vi "test.Template.vi"(8 "error in":errorcluster, 10 "Data":variant, 11 "Command":string) -> (0 "error out":errorcluster, 3 "Return Data":variant)   [LabVIEW 2014]
uses:
  Private/Class/meth.Constructor.vi
  Private/Class/meth.Destructor.vi
  GLue.lvlib
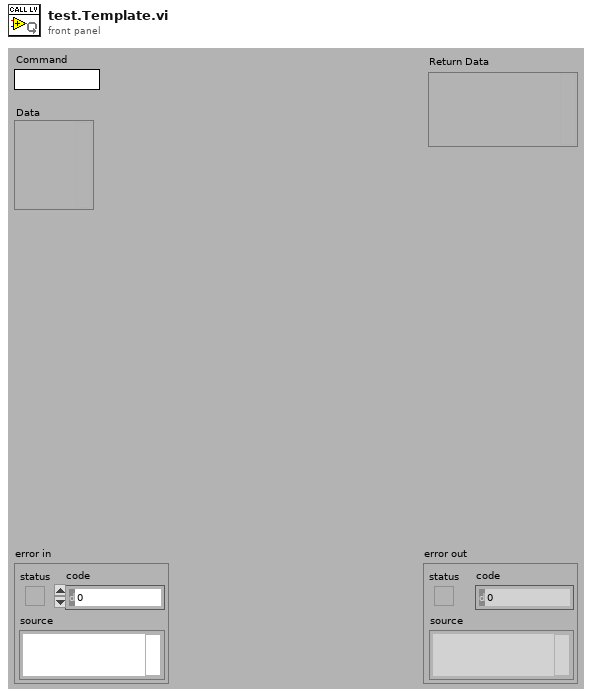
[diagram p1: front panel]
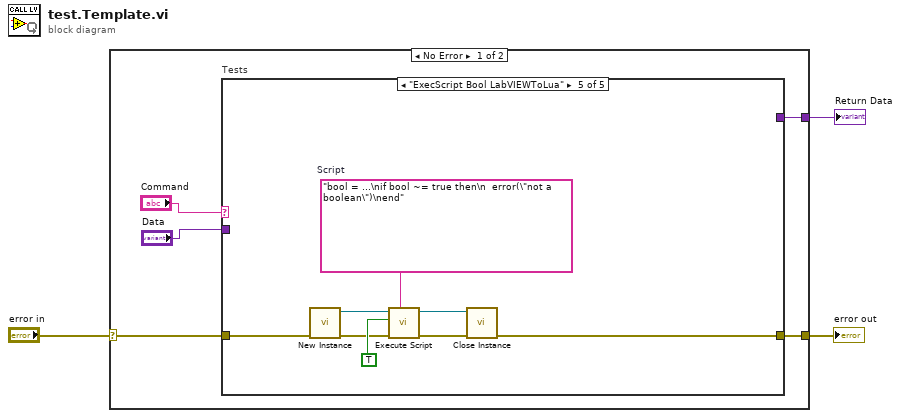
[diagram p0: block diagram]
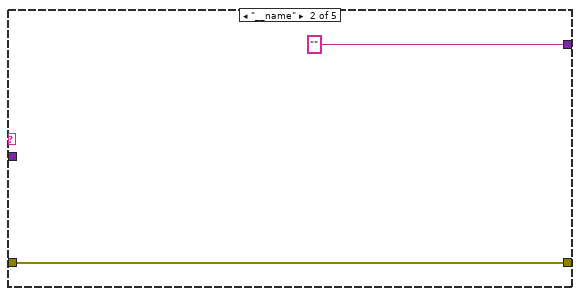
[diagram p3: hidden frame]
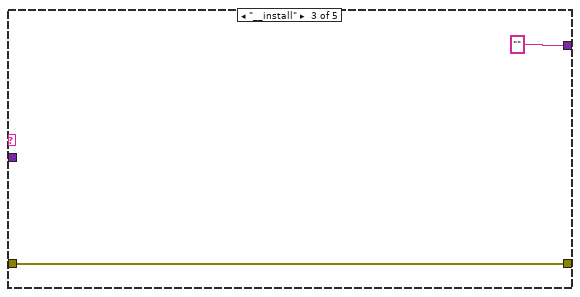
[diagram p4: hidden frame]
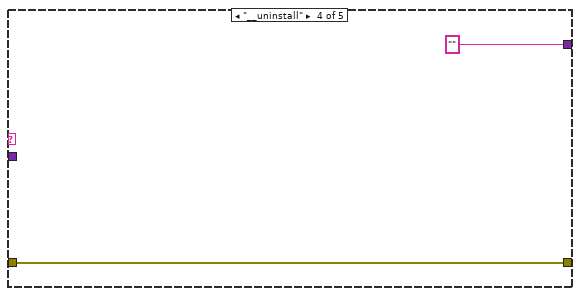
[diagram p5: hidden frame]
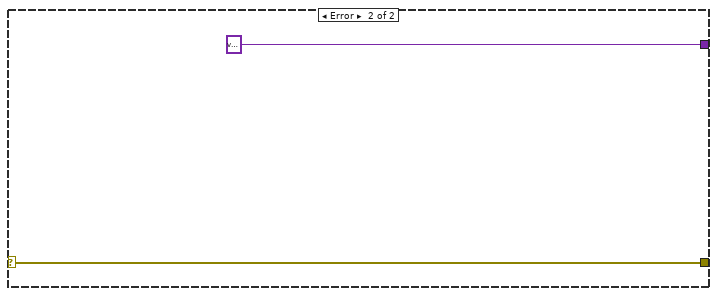
[diagram p6: hidden frame]
diagram:
  n1 = case shown="No Error" "error in" {
    selector: "error in" -> [w8 w26]
    tunnel: [w6 w26] -> w2
    tunnel: [w7 variant ("User Data")] -> w1
    frame No Error {
      n2 = case "Tests" shown="\"ExecScript Bool LabVIEWToLua\"" "Command" {
        tunnel: w8 -> [w10 w11 w13 w15 w18]
        tunnel: "Data" -> [w9 _ _ _ _]
        tunnel: [w9 "" "" "" _] -> w7
        tunnel: [w10 w11 w13 w15 w17] -> w6
        frame Default {
        }
        frame "__name" {
        }
        frame "__install" {
        }
        frame "__uninstall" {
        }
        frame "ExecScript Bool LabVIEWToLua" {
          w23 = "bool = ...\nif bool ~= true then\n  error(\"not a boolean\")\nend"  # Script
          n3 = call "New Instance.vi"("error in"=w18) -> ("error out"=w19:errorcluster, "GLue out"=w20:refnum<class "class.GLue.lvclass">)  [unwired: 9 in]
          n4 = call "Execute Script.vi"("Script"=w23, "error in"=w19, "Argument Data"=TRUE, "GLue in"=w20) -> ("error out"=w21:errorcluster, "GLue out"=w22:refnum<class "class.GLue.lvclass">)  [unwired: 5 in, 1 out]
          n5 = call "Close Instance.vi"("error in"=w21, "GLue in"=w22) -> ("error out"=w17:errorcluster)  [unwired: 9 in]
        }
      }
    }
    frame Error {
    }
  }
  "Return Data" <- w1
  "error out" <- w2
